vi "Element Factory.vi"(7 "VolatusAPI":refnum<class "VolatusAPI.lvclass">, 8 "error in (no error)":errorcluster, 9 "JSON":string, 10 "Ref":refnum<vi>, 11 "Element Type":string) -> (0 "error out":errorcluster, 2 "Is Indicator":bool, 3 "GUI Element":refnum<class "GUI Element.lvclass">)   [LabVIEW 2020, in "VolatusGUI.lvlib"]
uses:
  VolatusGUI.lvlib
  GUI Element/GUI Element.lvclass
  Volatus/VolatusAPI/VolatusAPI.lvclass
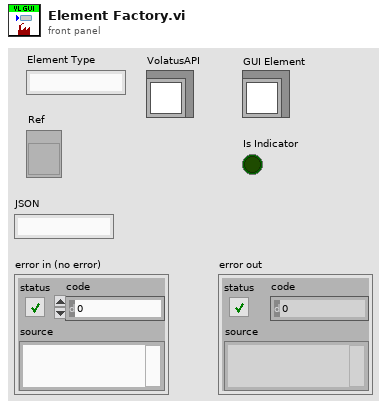
[diagram p1: front panel]
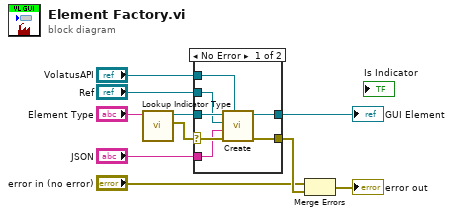
[diagram p0: block diagram]
diagram:
  n1 = call "Lookup Indicator Type.vi"("Element Type"="Element Type") -> ("error out"=w9:errorcluster, "Element"=w8:refnum<class "GUI Element.lvclass">)  [unwired: 9 in]
  n2 = case shown="No Error" w9 {
    selector: w9 -> [w16 w18]
    tunnel: w8 -> [w17 _]
    tunnel: "Ref" -> [w15 _]
    tunnel: "JSON" -> [w14 _]
    tunnel: [w13 w18] -> w4
    tunnel: [w12 _] -> w5
    tunnel: "VolatusAPI" -> [w11 _]
    frame No Error {
      n3 = call "Create.vi"("VolatusAPI"=w11, "error in (no error)"=w16, "JSON"=w14, "Ref"=w15, "GUI Element in"=w17) -> ("error out"=w13:errorcluster, "GUI Element out"=w12:refnum<class "GUI Element.lvclass">)  [unwired: 5 in]
    }
    frame Error {
    }
  }
  "GUI Element" <- w5
  n4 = Merge Errors("error in (no error)", w4) -> (→"error out":errorcluster)
